vi "WriteSendMsg2List.vi"(8 "发送通道":i32(ring) items=["CHN1", "CHN2", "CHN3", "CHN4", "CHN5", "CHN6", "CHN7", "CHN8", "CHN9", "CHN10", "CHN11", "CHN12", "CHN13", "CHN14", "CHN15", "CHN16", "CHN17", "CHN18", "CHN19", "CHN20", "CHN21", "CHN22", "CHN23", "CHN24", "CHN25", "CHN26", "CHN27", "CHN28", "CHN29", "CHN30", "CHN31", "CHN32"], 9 "SendOK":bool, 10 "CANframe":T1 {"ADLC" max=64; "AID" max=536870911}, 11 "Table输入":refnum<vi>) -> ()   [LabVIEW 2016]
uses:
  Ctrl/CAN_FrameInfo.ctl
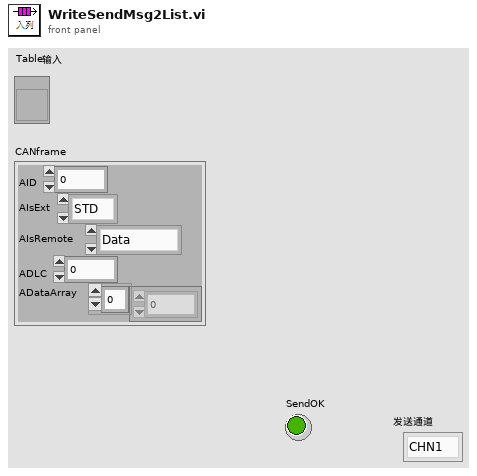
[diagram p1: front panel]
types:
  T1 = typedef "CAN_FrameInfo.ctl" = cluster{"AID":u32, "AIsExt":enum16{"STD", "EXT"}, "AIsRemote":enum16{"Data", "Remote"}, "ADLC":u8, "ADataArray":u8[]}
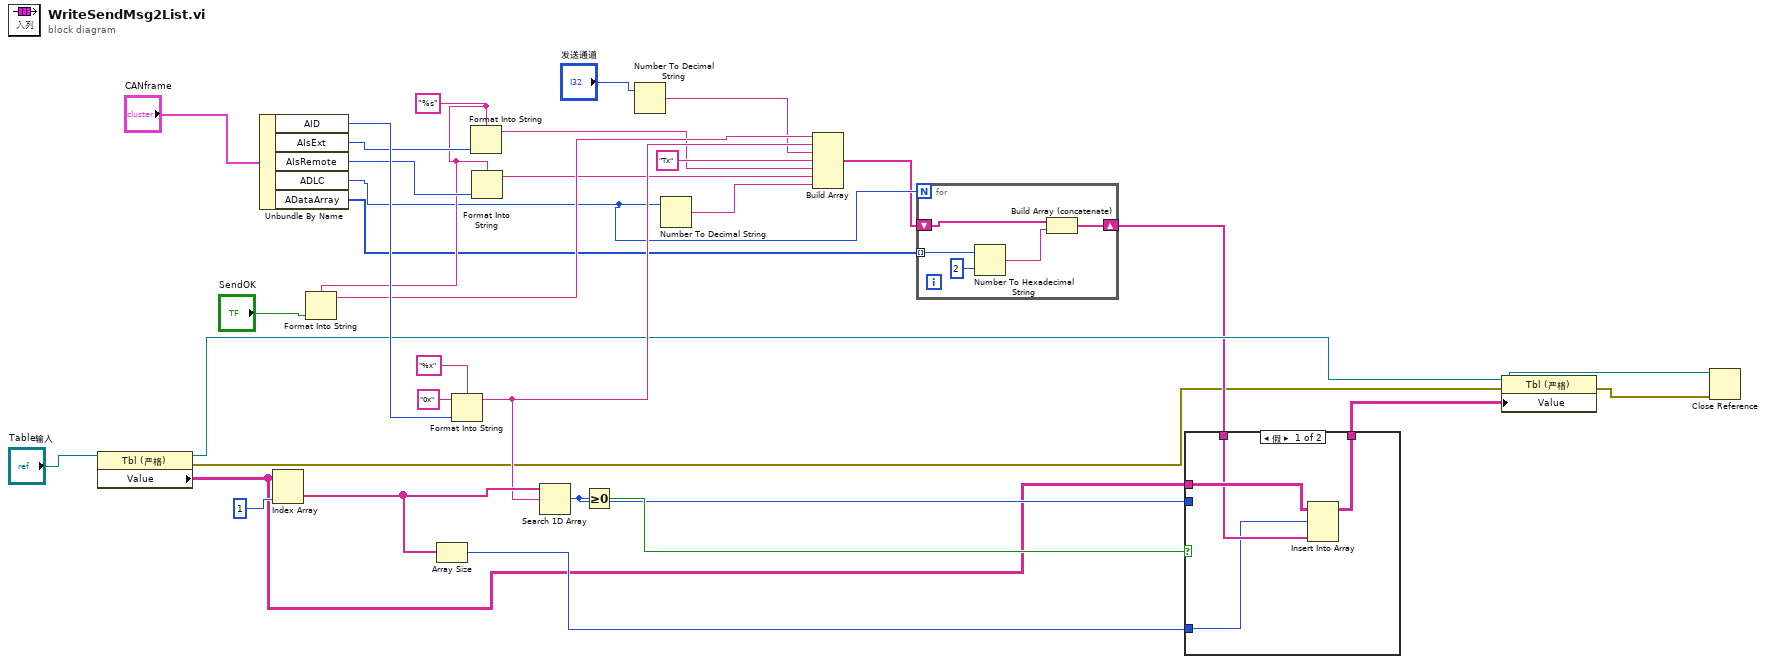
[diagram p0: block diagram]
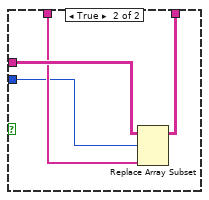
[diagram p2: hidden frame]
diagram:
  w19 = "%s" ("格式字符串")
  n1 = property class="Tbl (严格)"(reference="Table输入") -> (reference out=w7:refnum<vi>, error out=w1:errorcluster, "Value"=w4:string[][])  [unwired: 1 in]
  n2 = Unbundle By Name("CANframe") -> ("AID"=w30:u32, "AIsExt"=w22:enum16{"STD", "EXT"}, "AIsRemote"=w21:enum16{"Data", "Remote"}, "ADLC"=w10:u8, "ADataArray"=w9:u8[])
  n3 = Index Array(array=w4, index (col)=1 ("禁用的索引 (列)")) -> (element=w25:string[])  [unwired: 1 in]
  n4 = Format Into String(format string=w19, "SendOK") -> (resulting string=w18:string)  [unwired: 2 in, 1 out]
  n5 = Array Size(array=w25) -> (size(s)=w24:i32)
  n6 = Format Into String(format string="%x" ("格式字符串"), initial string="0x" ("初始字符串"), w30) -> (resulting string=w17:string)  [unwired: 1 in, 1 out]
  n7 = Format Into String(format string=w19, w22) -> (resulting string=w13:string)  [unwired: 2 in, 1 out]
  n8 = Format Into String(format string=w19, w21) -> (resulting string=w12:string)  [unwired: 2 in, 1 out]
  n9 = Search 1D Array(1D array=w25, element=w17) -> (index of element=w26:i32)  [unwired: 1 in]
  n10 = Greater Or Equal To 0?(x=w26) -> (x >= 0?=w27:bool)
  n11 = Number To Decimal String(number="发送通道") -> (decimal integer string=w15:string)  [unwired: 1 in]
  n12 = Number To Decimal String(number=w10) -> (decimal integer string=w11:string)  [unwired: 1 in]
  n13 = Build Array(w18, w17, w15, "Tx", w13, w12, w11) -> (w8:string[])
  n14 = for {
    N: w10 -> [_]
    tunnel: w9 -> [w37] mode=indexing
    shift-right: [w34] -> w3
    shift-left: w8 -> [w33]
    n15 = Number To Hexadecimal String(1:i16 2 ("宽度(-)"), 2:w37) -> (0:w35:string)
    n16 = Build Array (concatenate)(w33, w35) -> (w34:string[])
  }
  n17 = case shown="假" w27 {
    tunnel: w26 -> [_ w43]
    tunnel: w24 -> [w39 _]
    tunnel: w4 -> [w41 w45]
    tunnel: w3 -> [w40 w44]
    tunnel: [w38 w42] -> w2
    frame False {
      n18 = Insert Into Array(array=w41, index (row)=w39, new element=w40) -> (w38:string[][])  [unwired: 1 in]
    }
    frame True {
      n19 = Replace Array Subset(array=w45, new element=w44, index (row)=w43) -> (w42:string[][])  [unwired: 1 in]
    }
  }
  n20 = property class="Tbl (严格)"(reference=w7, error in=w1, "Value"=w2) -> (reference out=w6:refnum<vi>, error out=w5:errorcluster)
  n21 = Close Reference(reference=w6, error in (no error)=w5) -> ()  [unwired: 1 out]
